vi "Repack Color Array to Color.vi"(11 "Input Array U32x8":u32[](array[numeric])=[0, 0, 0, 0, 0, 0, 0, 0]) -> (3 "Colour Pixel Data":T1)   [LabVIEW 2020, in "NI_VDM_FPGA_Basics.lvlib"]
uses:
  <vilib>/visionFPGA/NI_VDM_FPGA_Basics.lvlib
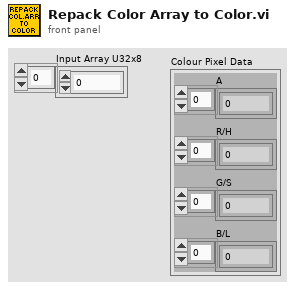
[diagram p1: front panel]
types:
  T1 = cluster{"A":u8[], "R/H":u8[], "G/S":u8[], "B/L":u8[]}
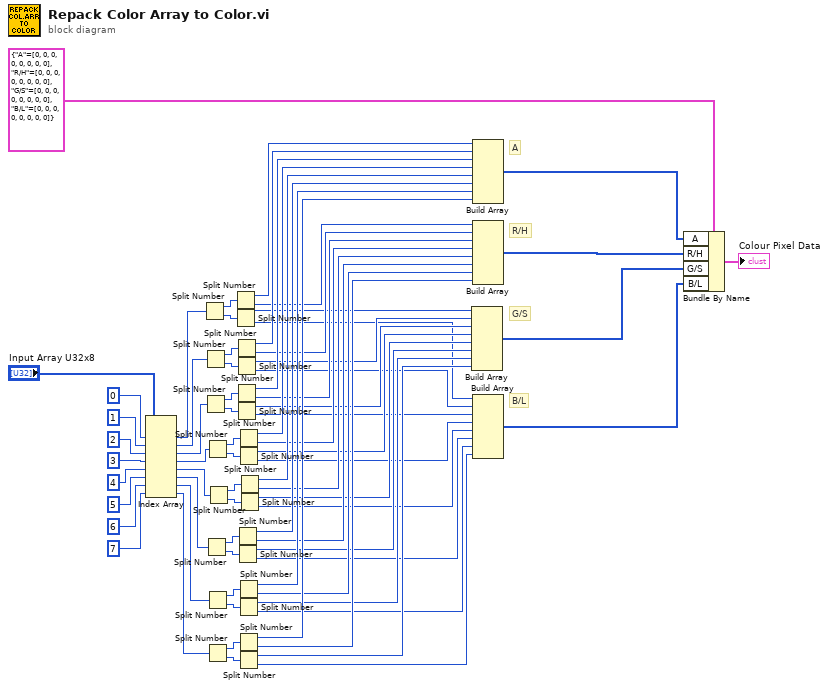
[diagram p0: block diagram]
diagram:
  # "B/L"
  # "G/S"
  # "R/H"
  # "A"
  n1 = Index Array(array="Input Array U32x8", index #1=0 ("index"), index #2=1 ("index"), index #3=2 ("index"), index #4=3 ("index"), index #5=4 ("index"), index #6=5 ("index"), index #7=6 ("index"), index #8=7 ("index")) -> (element #1=w62:u32, element #2=w53:u32, element #3=w52:u32, element #4=w51:u32, element #5=w48:u32, element #6=w45:u32, element #7=w42:u32, element #8=w39:u32)
  n2 = Split Number(x=w62) -> (hi(x)=w60:u16, lo(x)=w61:u16)
  n3 = Split Number(x=w53) -> (hi(x)=w59:u16, lo(x)=w58:u16)
  n4 = Split Number(x=w52) -> (hi(x)=w56:u16, lo(x)=w57:u16)
  n5 = Split Number(x=w45) -> (hi(x)=w47:u16, lo(x)=w46:u16)
  n6 = Split Number(x=w51) -> (hi(x)=w55:u16, lo(x)=w54:u16)
  n7 = Split Number(x=w42) -> (hi(x)=w43:u16, lo(x)=w44:u16)
  n8 = Split Number(x=w39) -> (hi(x)=w41:u16, lo(x)=w40:u16)
  n9 = Split Number(x=w48) -> (hi(x)=w49:u16, lo(x)=w50:u16)
  n10 = Split Number(x=w60) -> (hi(x)=w38:u8, lo(x)=w23:u8)
  n11 = Split Number(x=w61) -> (hi(x)=w21:u8, lo(x)=w7:u8)
  n12 = Split Number(x=w59) -> (hi(x)=w37:u8, lo(x)=w24:u8)
  n13 = Split Number(x=w58) -> (hi(x)=w22:u8, lo(x)=w8:u8)
  n14 = Split Number(x=w56) -> (hi(x)=w31:u8, lo(x)=w25:u8)
  n15 = Split Number(x=w57) -> (hi(x)=w20:u8, lo(x)=w9:u8)
  n16 = Split Number(x=w47) -> (hi(x)=w34:u8, lo(x)=w28:u8)
  n17 = Split Number(x=w46) -> (hi(x)=w17:u8, lo(x)=w12:u8)
  n18 = Split Number(x=w55) -> (hi(x)=w32:u8, lo(x)=w26:u8)
  n19 = Split Number(x=w54) -> (hi(x)=w19:u8, lo(x)=w10:u8)
  n20 = Split Number(x=w43) -> (hi(x)=w35:u8, lo(x)=w29:u8)
  n21 = Split Number(x=w44) -> (hi(x)=w16:u8, lo(x)=w13:u8)
  n22 = Split Number(x=w41) -> (hi(x)=w36:u8, lo(x)=w30:u8)
  n23 = Split Number(x=w40) -> (hi(x)=w15:u8, lo(x)=w14:u8)
  n24 = Split Number(x=w49) -> (hi(x)=w33:u8, lo(x)=w27:u8)
  n25 = Split Number(x=w50) -> (hi(x)=w18:u8, lo(x)=w11:u8)
  n26 = Build Array(w21, w22, w20, w19, w18, w17, w16, w15) -> (w3:u8[])
  n27 = Build Array(w38, w37, w31, w32, w33, w34, w35, w36) -> (w5:u8[])
  n28 = Build Array(w23, w24, w25, w26, w27, w28, w29, w30) -> (w4:u8[])
  n29 = Build Array(w7, w8, w9, w10, w11, w12, w13, w14) -> (w2:u8[])
  n30 = Bundle By Name(cluster=T1 {"A"=[0, 0, 0, 0, 0, 0, 0, 0], "R/H"=[0, 0, 0, 0, 0, 0, 0, 0], "G/S"=[0, 0, 0, 0, 0, 0, 0, 0], "B/L"=[0, 0, 0, 0, 0, 0, 0, 0]} ("Pixel Data"), "A"=w5, "R/H"=w4, "G/S"=w3, "B/L"=w2) -> (→"Colour Pixel Data":T1)
